vi "configuration class to editor name.vi"(7 "class type":T1, 8 "error in":errorcluster, 11 "configuration class name":string) -> (0 "error out":errorcluster, 3 "editor node class name":string)   [LabVIEW 2013, in "PL_class cache.lvlib"]
uses:
  PL_class cache.lvlib
  class type.ctl
  cache data.vi
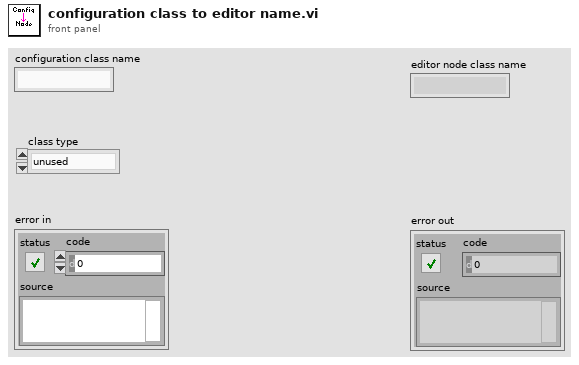
[diagram p1: front panel]
types:
  T1 = typedef "PL_class cache.lvlib/class type.ctl" = enum16{"unused", "target", "engine", "module"}
  T2 = typedef "PL_class cache.lvlib/cached class information.ctl" = cluster{"targets":T3[], "engines":T4[], "modules":T4[], "ignored class list":path[]}
  T3 = typedef "PL_class cache.lvlib/target class metadata.ctl" = cluster{"file name":string, "fully qualified name":string, "menu display name":string, "configuration class name":string}
  T4 = typedef "PL_class cache.lvlib/class metadata.ctl" = cluster{"file name":string, "fully qualified name":string, "menu display name":string, "configuration class":string, "instances allowed":i32, "supported targets":T5[]}
  T5 = typedef "TBM configuration.lvclass/Target Types.ctl" = enum16{"Windows", "Mac", "Linux", "Linux RT ARM", "VxWorks", "Pharlap", "Other", "Linux RT x64"}
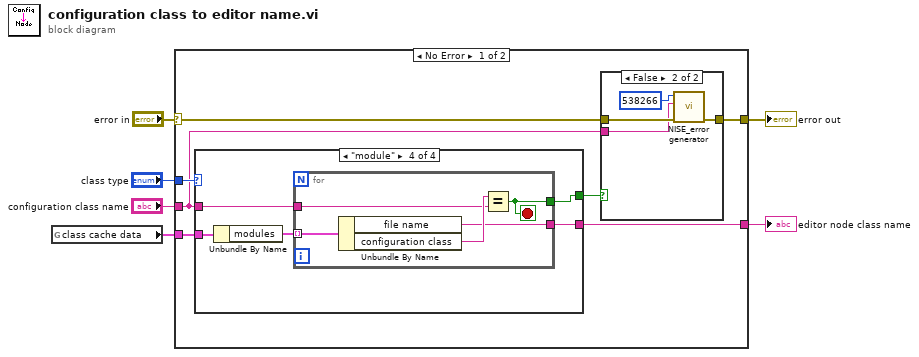
[diagram p0: block diagram]
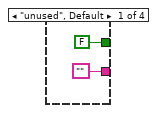
[diagram p2: hidden frame]
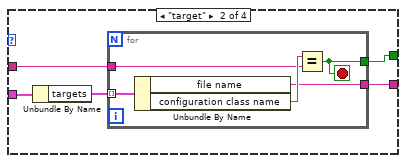
[diagram p3: hidden frame]
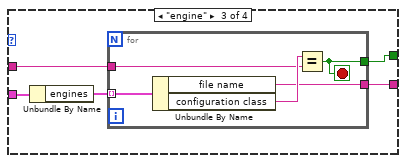
[diagram p4: hidden frame]
diagram:
  n1 = global read "cache data.vi" "class cache data"() -> (w2:T2)
  n2 = case shown="No Error" "error in" {
    selector: "error in" -> [w10 w51]
    tunnel: "configuration class name" -> [w7 _]
    tunnel: [w13 w51] -> w4
    tunnel: "class type" -> [w12 _]
    tunnel: w2 -> [w8 _]
    tunnel: [w9 _] -> w1
    frame No Error {
      n3 = case shown="\"module\"" w12 {
        tunnel: [FALSE w17 w27 w37] -> w11
        tunnel: ["" w16 w26 w36] -> w9
        tunnel: w8 -> [_ w20 w30 w40]
        tunnel: w7 -> [_ w18 w28 w38]
        frame "unused", Default {
        }
        frame "target" {
          n4 = Unbundle By Name(w20) -> ("targets"=w19:T3[])
          n5 = for {
            tunnel: w19 -> [w25] mode=indexing
            tunnel: w18 -> [w23]
            tunnel: [w22] -> w17
            tunnel: [w21] -> w16
            stop <- w22 stop-if-true
            n6 = Unbundle By Name(w25) -> ("file name"=w21:string, "configuration class name"=w24:string)
            n7 = Equal?(x=w24, y=w23) -> (x = y?=w22:bool)
          }
        }
        frame "engine" {
          n8 = Unbundle By Name(w30) -> ("engines"=w29:T4[])
          n9 = for {
            tunnel: w29 -> [w35] mode=indexing
            tunnel: w28 -> [w33]
            tunnel: [w32] -> w27
            tunnel: [w31] -> w26
            stop <- w32 stop-if-true
            n10 = Unbundle By Name(w35) -> ("file name"=w31:string, "configuration class"=w34:string)
            n11 = Equal?(x=w34, y=w33) -> (x = y?=w32:bool)
          }
        }
        frame "module" {
          n12 = Unbundle By Name(w40) -> ("modules"=w39:T4[])
          n13 = for {
            tunnel: w39 -> [w45] mode=indexing
            tunnel: w38 -> [w43]
            tunnel: [w42] -> w37
            tunnel: [w41] -> w36
            stop <- w42 stop-if-true
            n14 = Unbundle By Name(w45) -> ("file name"=w41:string, "configuration class"=w44:string)
            n15 = Equal?(x=w44, y=w43) -> (x = y?=w42:bool)
          }
        }
      }
      n16 = case shown="False" w11 {
        tunnel: [w46 w49] -> w13
        tunnel: w10 -> [w46 w48]
        tunnel: w7 -> [_ w47]
        frame True {
        }
        frame False {
          n17 = call <vilib>:"NISE_error generator.vi"("error in"=w48, "append error message"=w47, "error code (0)"=538266) -> ("error out"=w49:errorcluster)  [unwired: 6 in]
        }
      }
    }
    frame Error {
    }
  }
  "editor node class name" <- w1
  "error out" <- w4
